vi "Add Channel Group.vi"(8 "error in":errorcluster, 10 "group name":string="Channel Group", 11 "log file in":T1 format="%.0x") -> (0 "error out":errorcluster, 2 "channel group":T1 format="%.0x", 3 "log file out":T1 format="%.0x")   [LabVIEW 2027, in "Embedded Data Logger Scripting.lvlib"]
uses:
  Embedded Data Logger Scripting.lvlib
  <vilib>/NI VeriStand/Custom Device API/Custom Device Item Ref.ctl
  Shared/Constants.vi
  <vilib>/NI VeriStand/Custom Device API/Custom Device API.lvlib
  Shared/Embedded Data Logger Shared.lvlib
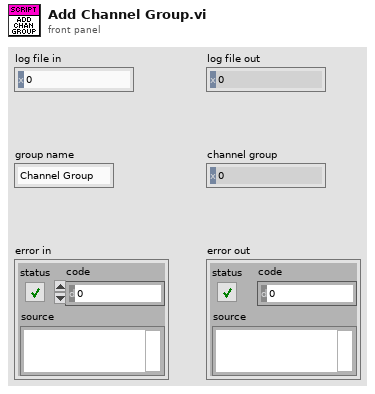
[diagram p1: front panel]
types:
  T1 = typedef "Custom Device API.lvlib/Custom Device Item Ref.ctl" = u64
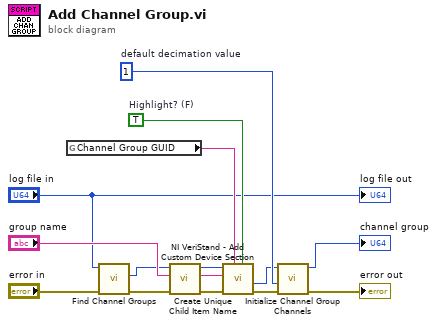
[diagram p0: block diagram]
diagram:
  w15 = 1  # default decimation value
  w9 = TRUE  # Highlight? (F)
  n1 = global read "Constants.vi" "Channel Group GUID"() -> (w11:string)
  n2 = call "Find Channel Groups.vi"("error in"="error in", "log file in"="log file in") -> ("error out"=w3:errorcluster, "channel groups"=w1:T1)  [unwired: 7 in, 1 out]
  n3 = call "Create Unique Child Item Name.vi"("error in (no error)"=w3, "Name in"="group name", "Parent Item Ref in"=w1) -> ("error out"=w6:errorcluster, "Unique Name out"=w8:string, "Parent Item Ref out"=w7:T1)  [unwired: 6 out]
  n4 = call <vilib>:"NI VeriStand - Add Custom Device Section.vi"("Highlight? (F)"=w9, "GUID (Default Section)"=w11, "error in (no error)"=w6, "Section Name"=w8, "Parent Ref in"=w7) -> ("error out"=w12:errorcluster, "Section Ptr"=w14:T1)  [unwired: 2 in, 3 out]
  n5 = call "Initialize Channel Group Channels.vi"("error in"=w12, "default decimation value"=w15, "channel group reference in"=w14) -> ("error out"=→"error out":errorcluster, "channel group reference out"=→"channel group":T1)  [unwired: 7 in]
  "log file out" <- "log file in"
